vi "Close Instrument Safely.vi"(8 "error in (no error)":errorcluster, 10 "Running (F)":bool, 11 "Optimizer Path":path) -> (0 "error out":errorcluster)   [LabVIEW 2020, in "Deep Reaction Optimizer Control Panel.lvlib" / "Instrument Manager.lvlib"]
doc: "Stops the pump if it is running, clears the character buffer on the pump, and closes the VISA resources given."
uses:
  process loops/Instrument Manager/Instrument Manager.lvlib
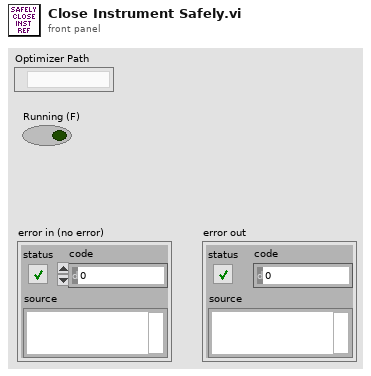
[diagram p1: front panel]
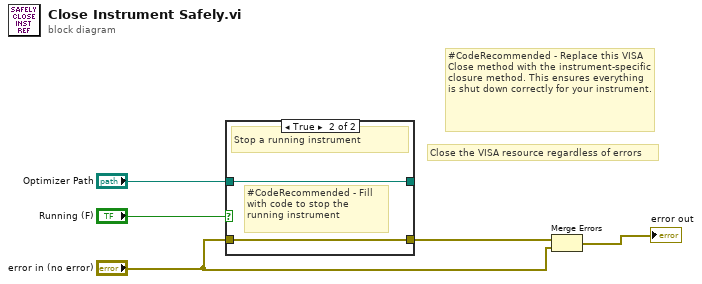
[diagram p0: block diagram]
diagram:
  # "#CodeRecommended - Replace this VISA Close method with the instrument-specific closure method. This ensures everything is shut down correctly for your instrument."
  # "Close the VISA resource regardless of errors"
  n1 = case shown="True" "Running (F)" {
    tunnel: "error in (no error)" -> [w7 w8]
    tunnel: [w7 w8] -> w1
    tunnel: "Optimizer Path" -> [w6 w9]
    tunnel: [w6 w9] -> _
    frame False {
    }
    frame True {
      # "#CodeRecommended - Fill with code to stop the\nrunning instrument"
      # "Stop a running instrument"
    }
  }
  n2 = Merge Errors(w1, "error in (no error)") -> (→"error out":errorcluster)
